vi "Write report.vi"(8 "error in (no error)":errorcluster, 11 "Boc12 in":refnum<class "Boc12.lvclass">) -> (0 "error out":errorcluster, 3 "Boc12 out":refnum<class "Boc12.lvclass">)   [LabVIEW 2017, in "Boc12.lvclass"]
uses:
  Boc12.lvclass
  home/andrew/projects/labview/boc/boc_setup/classes/report/Report.lvclass
  Report.lvclass/Report.ctl
  <vilib>/Utility/NIReport.llb/NI_report.lvclass
  Report.lvclass
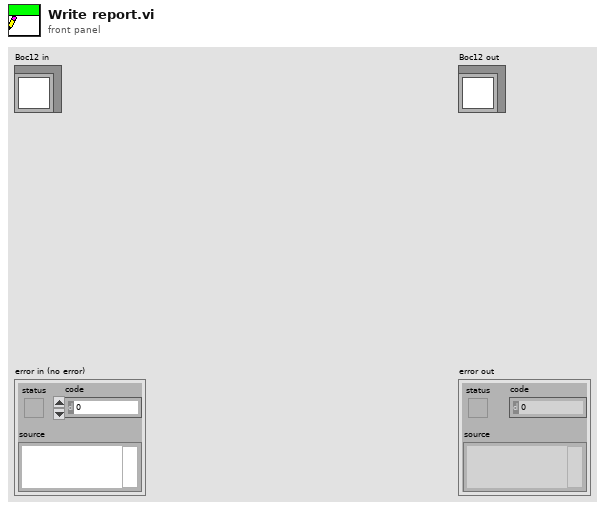
[diagram p1: front panel]
types:
  T1 = enum16{"maximized", "minimized", "normal", "no change"}
  T2 = enum16{"Standard Report", "HTML", "Word", "Excel"}
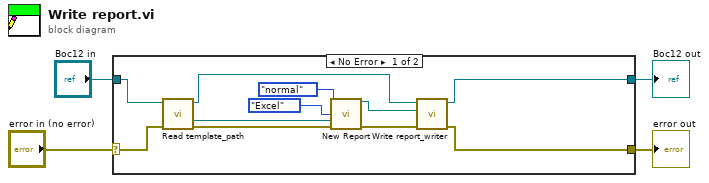
[diagram p0: block diagram]
diagram:
  n1 = case shown="No Error" "error in (no error)" {
    selector: "error in (no error)" -> [w12 w17]
    tunnel: "Boc12 in" -> [w14 w16]
    tunnel: [w6 w16] -> w3
    tunnel: [w5 w17] -> w2
    frame No Error {
      n2 = call "Read template_path.vi"("error in (no error)"=w12, "Report in"=w14) -> ("error out"=w10:errorcluster, "template_path"=w13:path, "Report out"=w7:refnum<class "Boc12.lvclass">)  [unwired: 7 in]
      n3 = call <vilib>:"New Report.vi"("window state (normal)"=T1."normal", "report type"=T2."Excel", "template (empty)"=w13, "error in (no error)"=w10) -> ("report out"=w9:refnum<class "NI_report.lvclass">, "error out"=w8:errorcluster)  [unwired: 10 in]
      n4 = call "Write report_writer.vi"("error in (no error)"=w8, "NI_report.lvclass"=w9, "Report in"=w7) -> ("error out"=w5:errorcluster, "Report out"=w6:refnum<class "Boc12.lvclass">)  [unwired: 7 in]
    }
    frame Error {
    }
  }
  "error out" <- w2
  "Boc12 out" <- w3
